vi "PICO init_2.vi"(10 "Mains Frequency":i16(ring) items=["50 Hz", "60 Hz"], 11 "Digital in":refnum<vi>) -> (2 "Handle":i16, 3 "Handle 2":i16)   [LabVIEW 2015]
uses:
  Program Files (x86)/Pico Technology/SDK/lib/usbtc08.dll
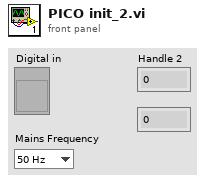
[diagram p1: front panel]
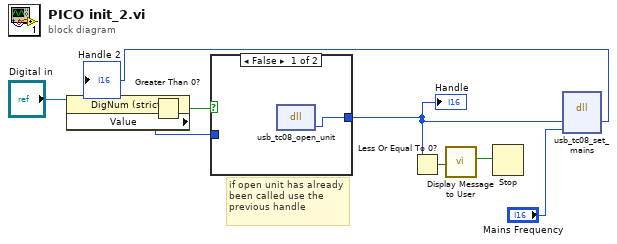
[diagram p0: block diagram]
diagram:
  # "if open unit has already been called use the previous handle"
  n1 = property class="DigNum (strict)"(reference="Digital in") -> ("Value"=w3:i16)  [unwired: 1 in, 2 out]
  n2 = Greater Than 0?(x=w3) -> (x > 0?=w2:bool)
  n3 = case shown="False" w2 {
    tunnel: [w9 w10] -> w5
    tunnel: w3 -> [_ w10]
    frame False {
      n4 = dll-call lib="C:/Program Files (x86)/Pico Technology/SDK/lib/usbtc08.dll" fn="usb_tc08_open_unit" label="OpenUnit"() -> ("Handle"=w9:i16)  [unwired: 3 in, 2 out]
    }
    frame True {
    }
  }
  "Handle" <- w5
  n5 = Less Or Equal To 0?(x=w5) -> (x <= 0?=w6:bool)
  n6 = call "Display Message to User"("Enable"=w6) -> ("OK"=w7:bool)  [unwired: 9 in, 1 out]
  n7 = Stop(stop? (T)=w7) -> ()
  n8 = dll-call lib="C:/Program Files (x86)/Pico Technology/SDK/lib/usbtc08.dll" fn="usb_tc08_set_mains" label="Set Mains"("Handle"=w5, "sixtyHertz"="Mains Frequency") -> ("Handle"=→"Handle 2":i16)  [unwired: 5 in, 2 out]
